vi "Test Assertion.vi"(11 "Test Case In":refnum<class "My Test.lvclass">) -> (0 "error out":errorcluster, 3 "Test Case Out":refnum<class "My Test.lvclass">)   [LabVIEW 2020, in "My Test.lvclass"]
uses:
  My Test.lvclass
  My Test.lvclass/My Test.ctl
  0369b00e-c90d-4403-a501-2e7f79e1a782.vi
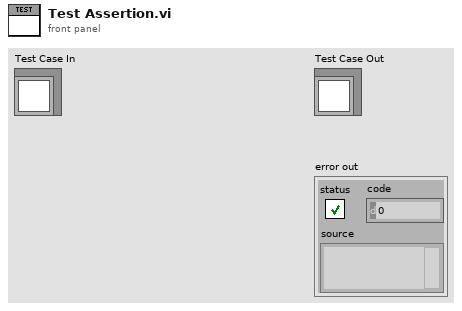
[diagram p1: front panel]
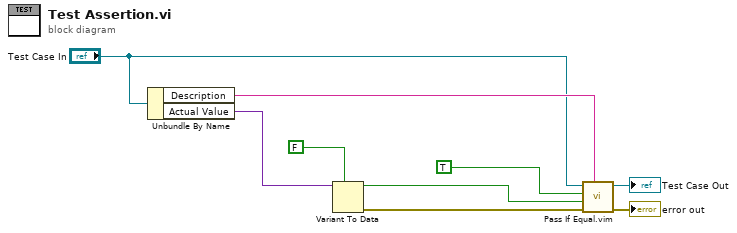
[diagram p0: block diagram]
diagram:
  n1 = Unbundle By Name("Test Case In") -> ("Description"=w3:string, "Actual Value"=w7:variant)
  n2 = Variant To Data(type=FALSE, Variant=w7) -> (data=w5:bool, error out=w2:errorcluster)  [unwired: 1 in]
  n3 = call "Pass If Equal.vim"("Description"=w3, "error in (no error)"=w2, "Actual"=w5, "Expected"=TRUE, "LUnit Test Case In"="Test Case In") -> ("error out"=→"error out":errorcluster, "LUnit Test Case Out"=→"Test Case Out":refnum<class "My Test.lvclass">)  [unwired: 5 in]
